vi "DllFxpAddTemp.vi"(6 "ready for output":bool, 8 "enable":bool, 9 "input valid":bool, 10 "y":fxp<+,16,1>, 11 "x":fxp<+,16,1>) -> (1 "output valid":bool, 2 "overflow?":bool, 3 "z":fxp<+,17,2> format="%.16g", 4 "ready for input":bool)   [LabVIEW 2017]
uses:
  <vilib>/rvi/FXPMathLib/FxpAdd/subVIs/nifxpmath_Add_SimConfig.ctl
  <vilib>/fxp/LVFixedPointQuantizationPolicyTypeDef.ctl
  <vilib>/fxp/LVFixedPointOverflowPolicyTypeDef.ctl
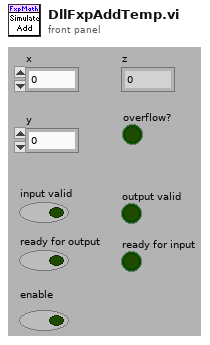
[diagram p1: front panel]
types:
  T1 = typedef "nifxpmath_Add_SimConfig.ctl" = cluster{"kXSigned":bool, "kXWl":u32, "kXIwl":i32, "kYSigned":bool, "kYWl":u32, "kYIwl":i32, "kZSigned":bool, "kZWl":u32, "kZIwl":i32, "Fixed-Point:Quantization Policy":T2, "Fixed-Point:Overflow Policy":T3, "OutputRegister":bool, "SupportSCTL?":bool, "kShowEnable":bool}
  T2 = typedef "LVFixedPointQuantizationPolicyTypeDef.ctl" = enum32{"Truncate", "Round-Half-Up (Asymmetric)", "Round-Half-Even"}
  T3 = typedef "LVFixedPointOverflowPolicyTypeDef.ctl" = enum32{"Wrap", "Saturate"}
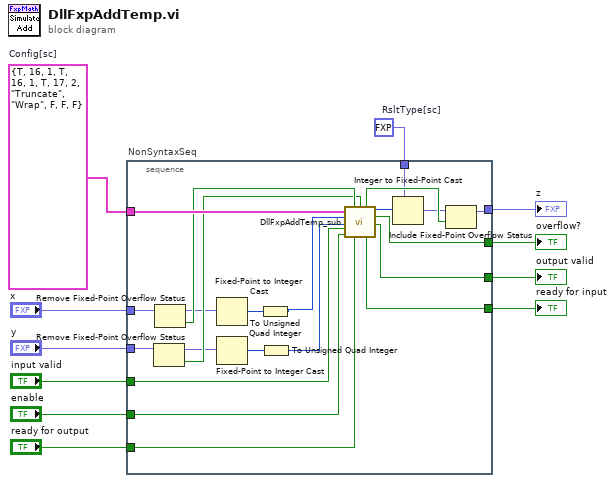
[diagram p0: block diagram]
diagram:
  w2 = T1 {"kXSigned"=TRUE, "kXWl"=16, "kXIwl"=1, "kYSigned"=TRUE, "kYWl"=16, "kYIwl"=1, "kZSigned"=TRUE, "kZWl"=17, "kZIwl"=2, "Fixed-Point:Quantization Policy"=enum."Truncate", "Fixed-Point:Overflow Policy"=enum."Wrap", "OutputRegister"=FALSE, "SupportSCTL?"=FALSE, "kShowEnable"=FALSE}  # Config[sc]
  w7 = fxp<+,17,2> 0.0  # RsltType[sc]
  n1 = stacked-sequence "NonSyntaxSeq" {
    tunnel: "x" -> [w27]
    tunnel: "y" -> [w25]
    tunnel: w7 -> [w13]
    tunnel: [w22] -> w6
    tunnel: "input valid" -> [w33]
    tunnel: [w32] -> w5
    tunnel: [w29] -> w3
    tunnel: [w28] -> w4
    tunnel: "ready for output" -> [w31]
    tunnel: w2 -> [w30]
    tunnel: "enable" -> [w21]
    frame #0 {
      n2 = Remove Fixed-Point Overflow Status(3:w25) -> (0:w24:bool, 1:w19:fxp<+,16,1>)
      n3 = Remove Fixed-Point Overflow Status(3:w27) -> (0:w26:bool, 1:w20:fxp<+,16,1>)
      n4 = Fixed-Point to Integer Cast(1:w20) -> (0:w17:u16)
      n5 = Fixed-Point to Integer Cast(1:w19) -> (0:w18:u16)
      n6 = To Unsigned Quad Integer(1:w17) -> (0:w16:u64)
      n7 = To Unsigned Quad Integer(1:w18) -> (0:w15:u64)
      n8 = call <vilib>:"DllFxpAddTemp_sub.vi"("Config[sc]"=w30, "x ovfl status"=w26, "y ovfl status"=w24, "x"=w16, "y"=w15, "input valid"=w33, "enable"=w21, "ready for output"=w31) -> ("z ovfl status"=w23:bool, "z"=w14:u64, "operational overflow"=w32:bool, "output valid"=w28:bool, "ready for input"=w29:bool)  [unwired: 3 out]
      n9 = Integer to Fixed-Point Cast(fixed-point type=w13, integer=w14) -> (fixed-point=w12:fxp<+,17,2>)
      n10 = Include Fixed-Point Overflow Status(2:w23, 3:w12) -> (1:w22:fxp<+,17,2>)
    }
  }
  "overflow?" <- w5
  "z" <- w6
  "output valid" <- w4
  "ready for input" <- w3
